vi "Disconnect.vi"(8 "error in (no error)":errorcluster, 11 "TCP_Client in":refnum<class "TCP_Client.lvclass">) -> (0 "error out":errorcluster, 3 "TCP_Client out":refnum<class "TCP_Client.lvclass">)   [LabVIEW 2018, in "TCP_Client.lvlib" / "TCP_Client.lvclass"]
uses:
  TCP_Client.lvclass
  TCP_Client.lvclass/TCP_Client.ctl
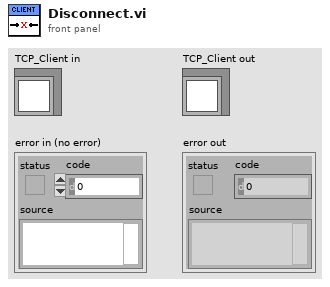
[diagram p1: front panel]
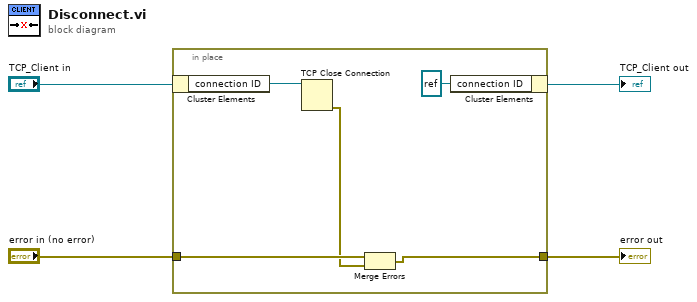
[diagram p0: block diagram]
diagram:
  n1 = in-place {
    in-place-border: "error in (no error)" -> [w7]
    in-place-border: [w5] -> w1
    n2 = in-place-cluster #1("TCP_Client in") -> ("connection ID"=w9:refnum<k5>)
    n3 = TCP Close Connection(connection ID=w9) -> (error out=w6:errorcluster)  [unwired: 2 in, 1 out]
    n4 = Merge Errors(w7, w6) -> (w5:errorcluster)
    n5 = in-place-cluster #1("connection ID"=refnum<k5> refnum) -> (→"TCP_Client out":refnum<class "TCP_Client.lvclass">)
  }
  "error out" <- w1
